vi "LWXPS_PositionerCompensationPhaseCorrectionFiltersGet.vi"(0 "XPS Reference IN":refnum<k24>, 2 "Positioner Name":string, 5 "LabVIEW error IN":errorcluster) -> (10 "XPS Reference OUT":refnum<k24>, 11 "LabVIEW error OUT":errorcluster, 12 "Returned error code":i32, 13 "XPS Error String":string, 14 "Numerator frequency 1":dbl, 15 "Denominator frequency 1":dbl, 16 "Phase Correction Gain 1":dbl, 17 "Numerator frequency 2":dbl, 18 "Denominator frequency 2":dbl, 19 "Phase Correction Gain 2":dbl)   [LabVIEW 2014]
uses:
  D:/XPSQ8_LabView_Library/Development/Source/Dll/Newport.XPS.CommandInterface.dll
  Dll/Newport.XPS.CommandInterface.dll
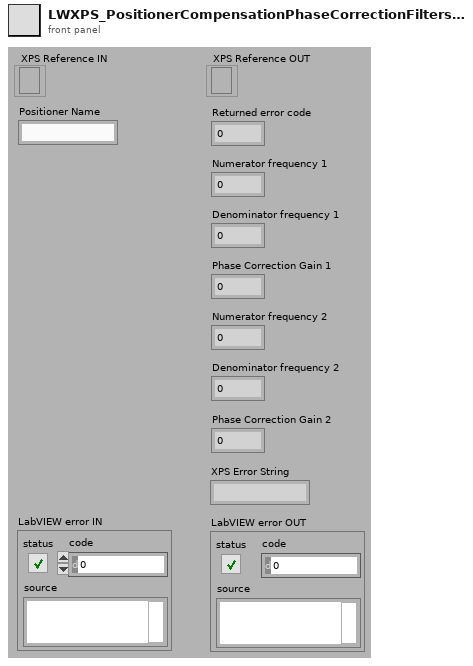
[diagram p1: front panel]
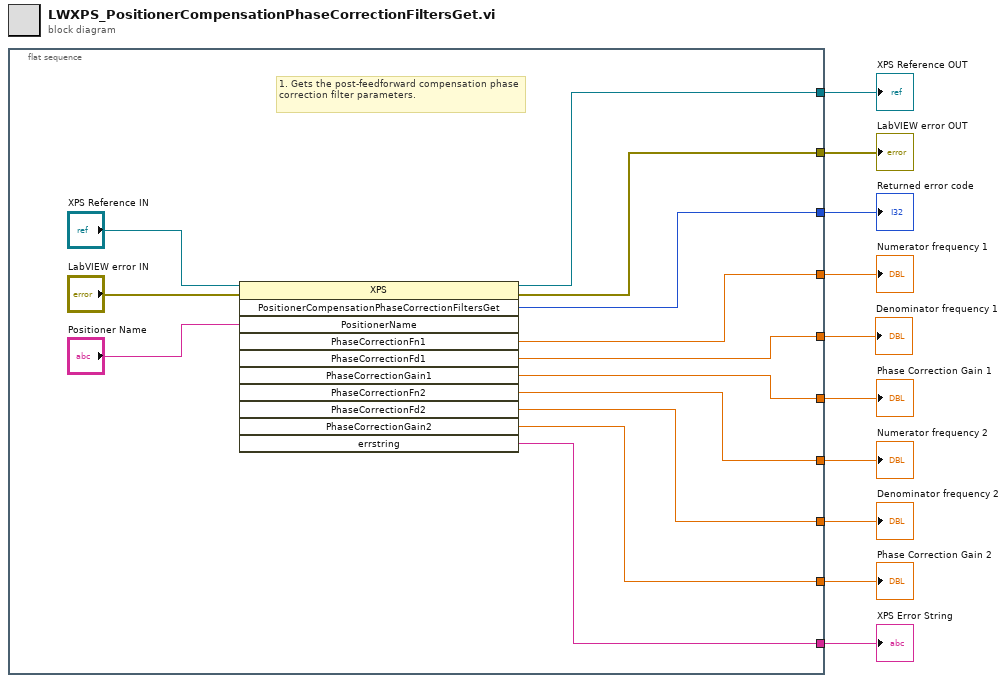
[diagram p0: block diagram]
diagram:
  n1 = flat-sequence {
    tunnel: [w21] -> w10
    tunnel: [w14] -> w9
    tunnel: [w22] -> w8
    tunnel: [w18] -> w7
    tunnel: [w17] -> w6
    tunnel: [w15] -> w5
    tunnel: [w16] -> w3
    tunnel: [w13] -> w2
    tunnel: [w12] -> w4
    tunnel: [w11] -> w1
    frame #0 {
      # "1. Gets the post-feedforward compensation phase correction filter parameters."
      n2 = invoke class="XPS" method="PositionerCompensationPhaseCorrectionFiltersGet"(reference="XPS Reference IN", error in="LabVIEW error IN", "PositionerName"="Positioner Name") -> (reference out=w21:refnum<k24>, error out=w14:errorcluster, "PositionerCompensationPhaseCorrectionFiltersGet"=w22:i32, "PhaseCorrectionFn1"=w12:dbl, "PhaseCorrectionFd1"=w18:dbl, "PhaseCorrectionGain1"=w17:dbl, "PhaseCorrectionFn2"=w15:dbl, "PhaseCorrectionFd2"=w16:dbl, "PhaseCorrectionGain2"=w13:dbl, "errstring"=w11:string)  [unwired: 8 in, 1 out]
    }
  }
  "XPS Error String" <- w1
  "XPS Reference OUT" <- w10
  "LabVIEW error OUT" <- w9
  "Returned error code" <- w8
  "Denominator frequency 1" <- w7
  "Phase Correction Gain 1" <- w6
  "Numerator frequency 2" <- w5
  "Numerator frequency 1" <- w4
  "Denominator frequency 2" <- w3
  "Phase Correction Gain 2" <- w2
